vi "get primary NIC IP address and MAC.vi"(8 "error in":errorcluster, 11 "system session":refnum<k21>) -> (0 "error out":errorcluster, 2 "MAC address":string, 3 "IP address":string)   [LabVIEW 2014, in "SMI.lvlib" / "Device.lvclass"]
uses:
  Device.lvclass
  <vilib>/nisyscfg/Find Hardware.vi
  <vilib>/nisyscfg/Close (Hardware).vi
  <vilib>/nisyscfg/Close (System).vi
  <vilib>/nisyscfg/nisyscfg.lvlib
  <resource>/objmgr/niflexriosae.rc
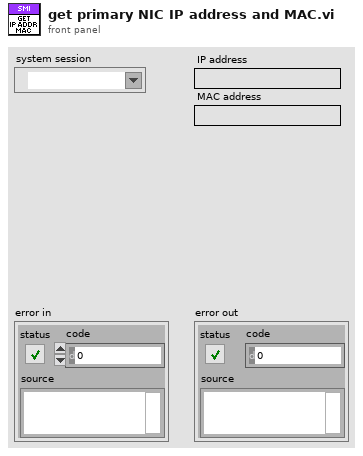
[diagram p1: front panel]
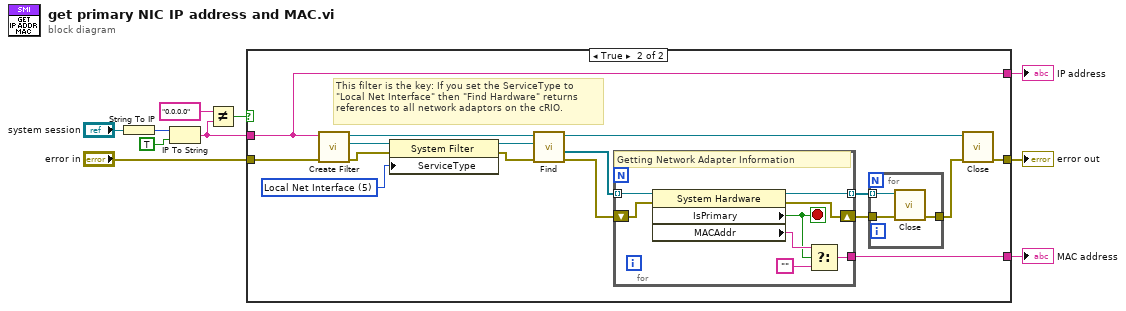
[diagram p0: block diagram]
diagram:
  n1 = String To IP(1:"system session") -> (0:w5:u32)
  n2 = IP To String(1:TRUE ("dot notation? (F)"), 2:w5) -> (0:w2:string)
  n3 = Not Equal?(x="0.0.0.0" ("y"), y=w2) -> (x != y?=w3:bool)
  n4 = case shown="True" w3 {
    tunnel: "error in" -> [w11 w27]
    tunnel: [w11 w26] -> w9
    tunnel: [_ w25] -> w8
    tunnel: w2 -> [_ w12]
    tunnel: [_ w12] -> w1
    frame False {
    }
    frame True {
      w19 = u32 5 items=["NI Network Resource", "NI Real-Time", "NI System Configuration", "NI Web Interface", "Local System", "Local Net Interface", "Local Time Keeper", "Local Time Reference", "LXI Instrument"] ("Service Type")
      # "This filter is the key: If you set the ServiceType to\n\"Local Net Interface\" then \"Find Hardware\" returns\nreferences to all network adaptors on the cRIO."
      n5 = call <vilib>:"Create Filter.vi"("error in (no error)"=w27, "Session in"=w12) -> ("error out"=w22:errorcluster, "Filter out"=w18:refnum<k20>, "Session out"=w17:refnum<k21>)  [unwired: 7 in]
      n6 = property class="System Filter"(reference=w18, error in=w22, "ServiceType"=w19) -> (reference out=w20:refnum<k20>, error out=w21:errorcluster)
      n7 = call-poly <vilib>:"Find.vi"("error in (no error)"=w21, "Filter in"=w20, "Session in"=w17) -> ("error out"=w23:errorcluster, "Resources out"=w15:refnum<k20>[], "Session out"=w14:refnum<k21>)  [unwired: 5 in, 1 out]
      n8 = for {
        tunnel: w15 -> [w28] mode=indexing
        shift-right: [w33] -> w24
        shift-left: w23 -> [w35]
        tunnel: [w34] -> w16 mode=indexing
        tunnel: [w31] -> w25
        stop <- w29 stop-if-true
        # "Getting Network Adapter Information"
        n9 = property class="System Hardware"(reference=w28, error in=w35) -> (reference out=w34:refnum<k20>, error out=w33:errorcluster, "IsPrimary"=w29:bool, "MACAddr"=w32:string)
        n10 = Select(t=w32, s=w29, f="") -> (s? t:f=w31:string)
      }
      n11 = for {
        tunnel: [w38] -> w13
        tunnel: w24 -> [w37]
        tunnel: w16 -> [w36] mode=indexing
        n12 = call-poly <vilib>:"Close.vi"("error in (no error)"=w37, "Resource in"=w36) -> ("error out"=w38:errorcluster)  [unwired: 9 in]
      }
      n13 = call-poly <vilib>:"Close.vi"("error in (no error)"=w13, "Session in"=w14) -> ("error out"=w26:errorcluster)  [unwired: 9 in]
    }
  }
  "error out" <- w9
  "IP address" <- w1
  "MAC address" <- w8
